vi "Agilent VNA Convert Formated Data.vi"(7 "Display Format":T1, 10 "Number":cdb) -> (2 "Number":cdb)   [LabVIEW 2011]
uses:
  tests/S Parameter/TypeDefs/SP Measurement Format.ctl
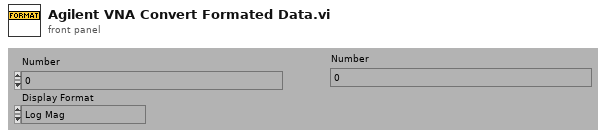
[diagram p1: front panel]
types:
  T1 = typedef "SP Measurement Format.ctl" = enum32{"Log Mag", "Phase", "Delay", "Smith (R+jX)", "Polar (Re/Im)", "Linear Mag", "SWR", "Real", "Imaginary", "Smith (Lin/Phase)", "Smith (Log/Phase)", "Smith (Real/Imag)", "Smith (G+jB)", "Polar (Lin/Phase)", "Polar (Log/Phase)", "Expanded Phase", "Positive Phase", "Inverted Smith", "Unwrapped Phase", "Power Out", "Power In", "Linear Mag/Phase", "Log Mag/Phase", "Real/Imaginary"}
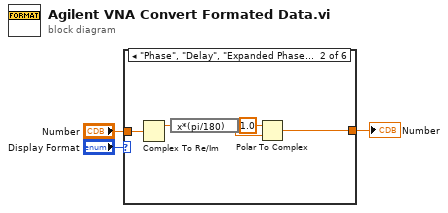
[diagram p0: block diagram]
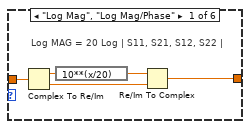
[diagram p2: hidden frame]
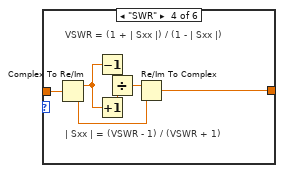
[diagram p4: hidden frame]
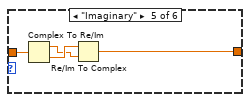
[diagram p5: hidden frame]
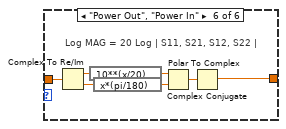
[diagram p6: hidden frame]
diagram:
  n1 = case shown="\"Phase\", \"Delay\", \"Expanded Phase\", \"Positive Phase\", \"Unwrapped Phase\"" "Display Format" {
    tunnel: [w5 w12 w14 w18 w22 w26] -> w2
    tunnel: "Number" -> [w4 w13 w14 w19 w25 w27]
    frame "Log Mag", "Log Mag/Phase" {
      # "Log MAG = 20 Log | S11, S21, S12, S22 |"
      n2 = Complex To Re/Im(x + iy=w4) -> (x=w7:dbl, y=w6:dbl)
      n3 = expression code="10**(x/20)"(w7) -> (w8:dbl)
      n4 = Re/Im To Complex(1:w6, 2:w8) -> (0:w5:cdb)
    }
    frame "Phase", "Delay", "Expanded Phase", "Positive Phase", "Unwrapped Phase" {
      n5 = Complex To Re/Im(x + iy=w13) -> (x=w11:dbl)  [unwired: 1 out]
      n6 = expression code="x*(pi/180)"(w11) -> (w10:dbl)
      n7 = Polar To Complex(1:w10, 2:1.0 ("r")) -> (0:w12:cdb)
    }
    frame "Smith (R+jX)".."Linear Mag", "Real", "Smith (Lin/Phase)".."Polar (Log/Phase)", "Inverted Smith", "Linear Mag/Phase", "Real/Imaginary" {
    }
    frame "SWR" {
      # "| Sxx | = (VSWR - 1) / (VSWR + 1)"
      # "VSWR = (1 + | Sxx |) / (1 - | Sxx |)"
      n8 = Complex To Re/Im(x + iy=w19) -> (x=w16:dbl, y=w15:dbl)
      n9 = Decrement(x=w16) -> (x-1=w21:dbl)
      n10 = Increment(x=w16) -> (x+1=w20:dbl)
      n11 = Divide(x=w21, y=w20) -> (x/y=w17:dbl)
      n12 = Re/Im To Complex(1:w15, 2:w17) -> (0:w18:cdb)
    }
    frame "Imaginary" {
      n13 = Complex To Re/Im(x + iy=w25) -> (x=w23:dbl, y=w24:dbl)
      n14 = Re/Im To Complex(1:w23, 2:w24) -> (0:w22:cdb)
    }
    frame "Power Out", "Power In" {
      # "Log MAG = 20 Log | S11, S21, S12, S22 |"
      n15 = Complex To Re/Im(x + iy=w27) -> (x=w28:dbl, y=w29:dbl)
      n16 = expression code="10**(x/20)"(w28) -> (w30:dbl)
      n17 = expression code="x*(pi/180)"(w29) -> (w31:dbl)
      n18 = Polar To Complex(1:w31, 2:w30) -> (0:w32:cdb)
      n19 = Complex Conjugate(1:w32) -> (0:w26:cdb)
    }
  }
  "Number" <- w2
